vi "psp_zeromq_send.vi"(1 "socket out":refnum<class "zmq_socket.lvclass">, 2 "archive":T1) -> (0 "error out":errorcluster)   [LabVIEW 2020]
uses:
  <vilib>/addons/zeromq/zmq_socket.lvclass
  archive_elyse/archive.ctl
  archive_elyse/sync_type_def.ctl
  archive_elyse/HT_type-def.ctl
  archive_elyse/HF_type_def.ctl
  archive_elyse/vacuum_type_def.ctl
  archive_elyse/modulator_type_def.ctl
  archive_elyse/water_cooling_type_def.ctl
  archive_elyse/all_magnets_type_def.ctl
panel:
  out "JSON string":string
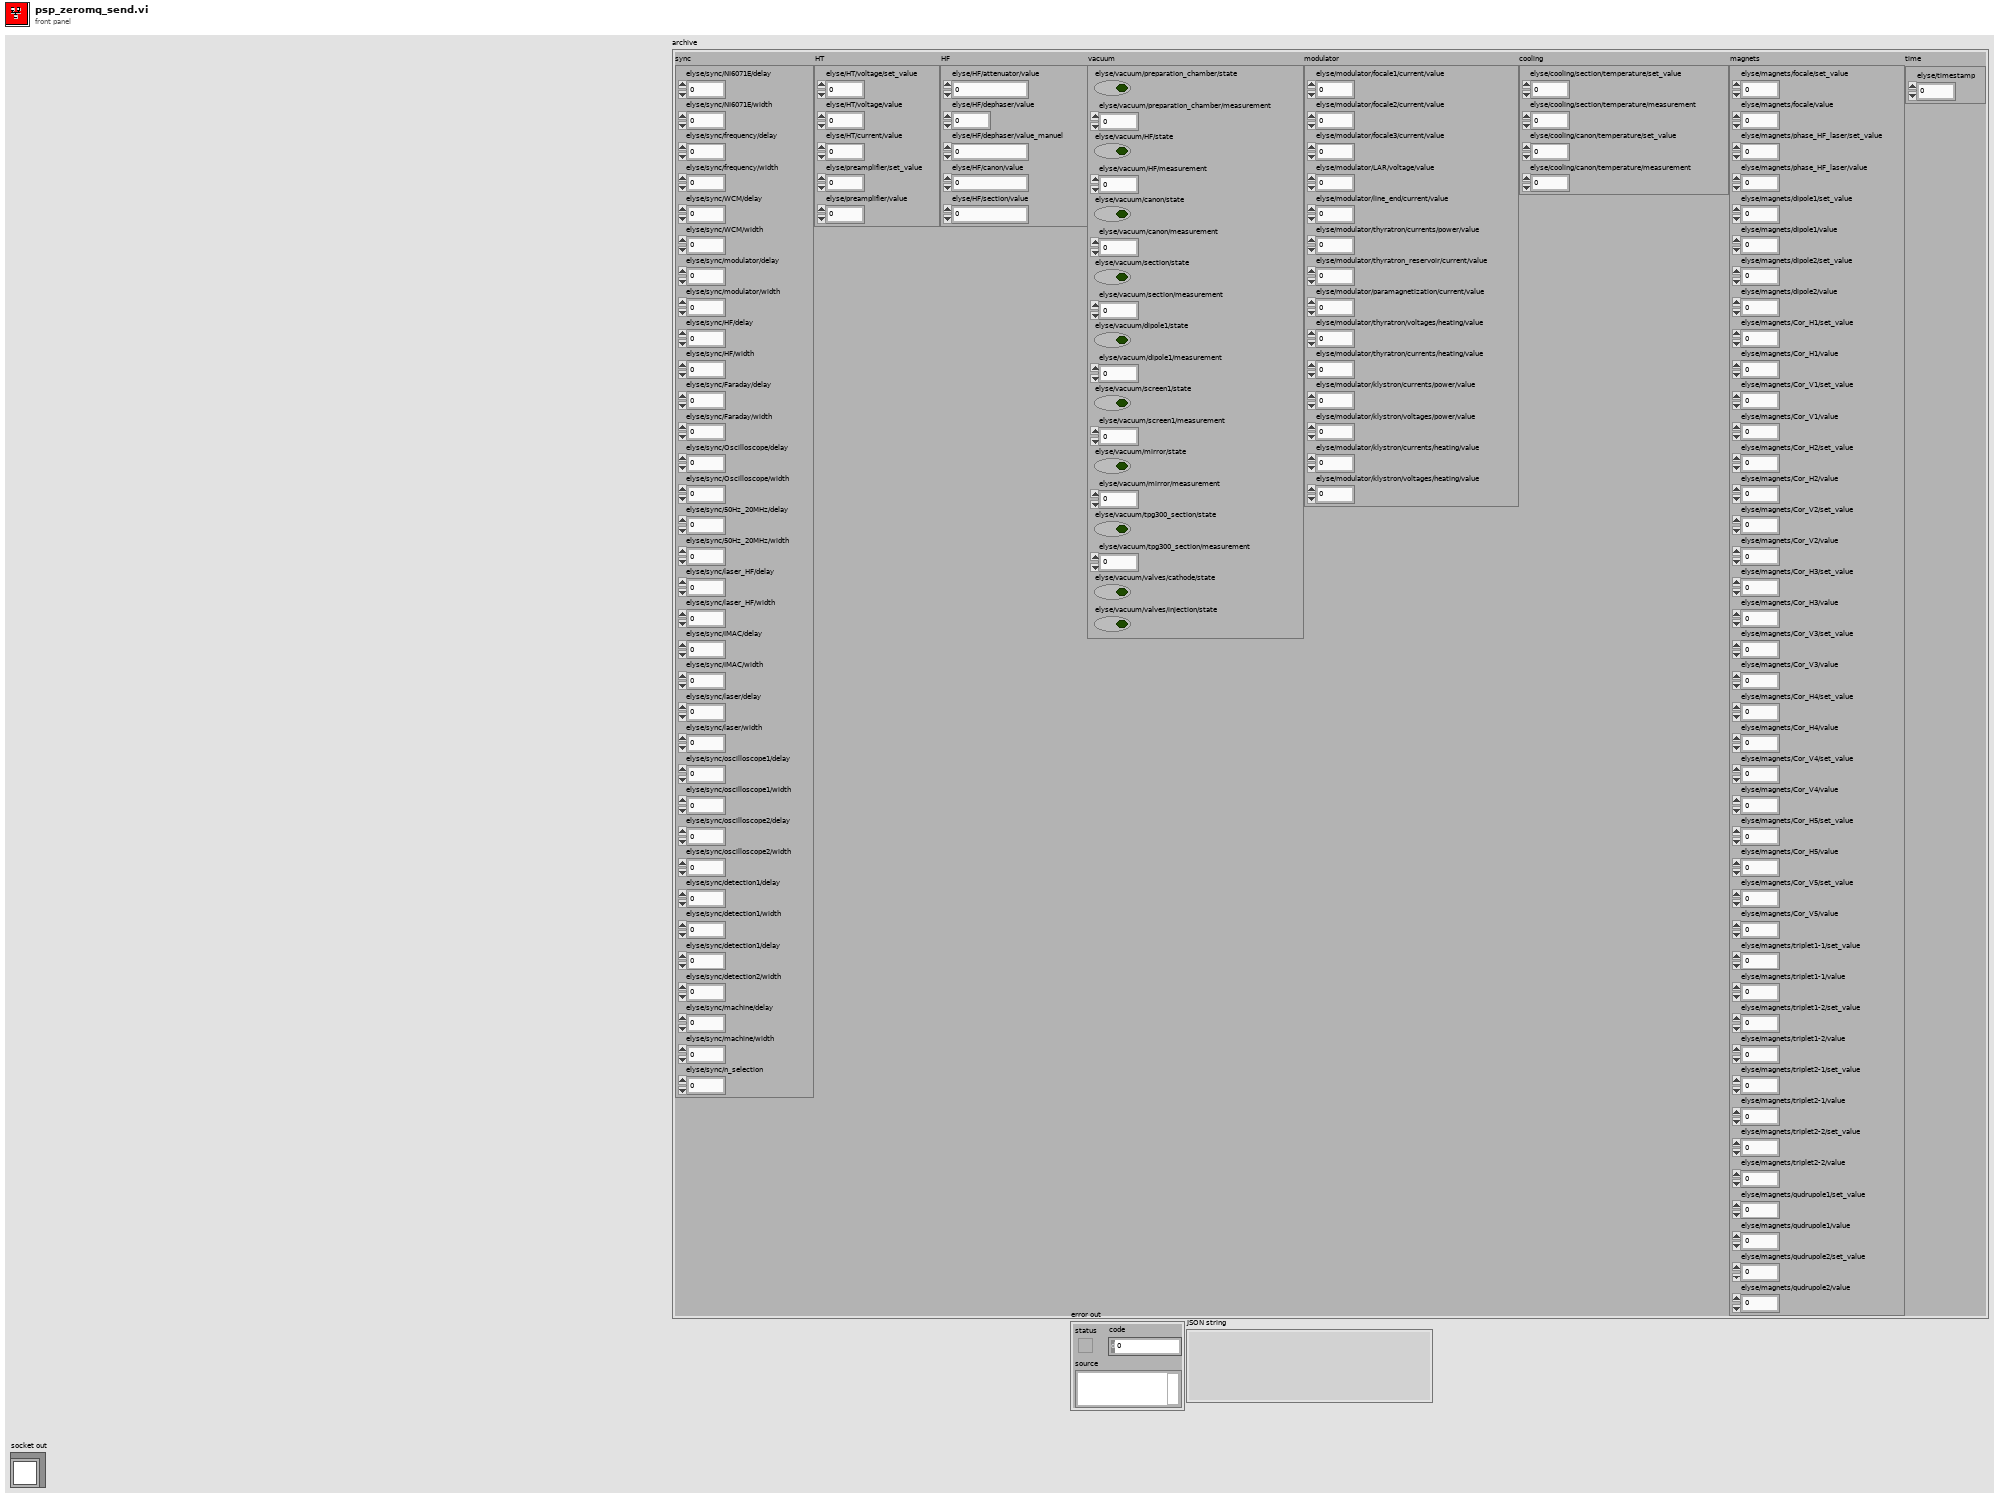
[diagram p1: front panel]
types:
  T1 = typedef "archive.ctl" = cluster{"sync":T2, "HT":T3, "HF":T4, "vacuum":T5, "modulator":T6, "cooling":T7, "magnets":T8, "time":cluster{"elyse/timestamp":dbl}}
  T2 = typedef "sync_type_def.ctl" = cluster{"elyse/sync/NI6071E/delay":dbl, "elyse/sync/NI6071E/width":dbl, "elyse/sync/frequency/delay":dbl, "elyse/sync/frequency/width":dbl, "elyse/sync/WCM/delay":dbl, "elyse/sync/WCM/width":dbl, "elyse/sync/modulator/delay":dbl, "elyse/sync/modulator/width":dbl, "elyse/sync/HF/delay":dbl, "elyse/sync/HF/width":dbl, "elyse/sync/Faraday/delay":dbl, "elyse/sync/Faraday/width":dbl, "elyse/sync/Oscilloscope/delay":dbl, "elyse/sync/Oscilloscope/width":dbl, "elyse/sync/50Hz_20MHz/delay":dbl, "elyse/sync/50Hz_20MHz/width":dbl, "elyse/sync/laser_HF/delay":dbl, "elyse/sync/laser_HF/width":dbl, "elyse/sync/IMAC/delay":dbl, "elyse/sync/IMAC/width":dbl, "elyse/sync/laser/delay":dbl, "elyse/sync/laser/width":dbl, "elyse/sync/oscilloscope1/delay":dbl, "elyse/sync/oscilloscope1/width":dbl, "elyse/sync/oscilloscope2/delay":dbl, "elyse/sync/oscilloscope2/width":dbl, "elyse/sync/detection1/delay":dbl, "elyse/sync/detection1/width":dbl, "elyse/sync/detection1/delay":dbl, "elyse/sync/detection2/width":dbl, "elyse/sync/machine/delay":dbl, "elyse/sync/machine/width":dbl, "elyse/sync/n_selection":dbl}
  T3 = typedef "HT_type-def.ctl" = cluster{"elyse/HT/voltage/set_value":dbl, "elyse/HT/voltage/value":dbl, "elyse/HT/current/value":dbl, "elyse/preamplifier/set_value":dbl, "elyse/preamplifier/value":dbl}
  T4 = typedef "HF_type_def.ctl" = cluster{"elyse/HF/attenuator/value":dbl, "elyse/HF/dephaser/value":dbl, "elyse/HF/dephaser/value_manuel":dbl, "elyse/HF/canon/value":dbl, "elyse/HF/section/value":dbl}
  T5 = typedef "vacuum_type_def.ctl" = cluster{"elyse/vacuum/preparation_chamber/state":bool, "elyse/vacuum/preparation_chamber/measurement":dbl, "elyse/vacuum/HF/state":bool, "elyse/vacuum/HF/measurement":dbl, "elyse/vacuum/canon/state":bool, "elyse/vacuum/canon/measurement":dbl, "elyse/vacuum/section/state":bool, "elyse/vacuum/section/measurement":dbl, "elyse/vacuum/dipole1/state":bool, "elyse/vacuum/dipole1/measurement":dbl, "elyse/vacuum/screen1/state":bool, "elyse/vacuum/screen1/measurement":dbl, "elyse/vacuum/mirror/state":bool, "elyse/vacuum/mirror/measurement":dbl, "elyse/vacuum/tpg300_section/state":bool, "elyse/vacuum/tpg300_section/measurement":dbl, "elyse/vacuum/valves/cathode/state":bool, "elyse/vacuum/valves/injection/state":bool}
  T6 = typedef "modulator_type_def.ctl" = cluster{"elyse/modulator/focale1/current/value":dbl, "elyse/modulator/focale2/current/value":dbl, "elyse/modulator/focale3/current/value":dbl, "elyse/modulator/LAR/voltage/value":dbl, "elyse/modulator/line_end/current/value":dbl, "elyse/modulator/thyratron/currents/power/value":dbl, "elyse/modulator/thyratron_reservoir/current/value":dbl, "elyse/modulator/paramagnetization/current/value":dbl, "elyse/modulator/thyratron/voltages/heating/value":dbl, "elyse/modulator/thyratron/currents/heating/value":dbl, "elyse/modulator/klystron/currents/power/value":dbl, "elyse/modulator/klystron/voltages/power/value":dbl, "elyse/modulator/klystron/currents/heating/value":dbl, "elyse/modulator/klystron/voltages/heating/value":dbl}
  T7 = typedef "water_cooling_type_def.ctl" = cluster{"elyse/cooling/section/temperature/set_value":dbl, "elyse/cooling/section/temperature/measurement":dbl, "elyse/cooling/canon/temperature/set_value":dbl, "elyse/cooling/canon/temperature/measurement":dbl}
  T8 = typedef "all_magnets_type_def.ctl" = cluster{"elyse/magnets/focale/set_value":dbl, "elyse/magnets/focale/value":dbl, "elyse/magnets/phase_HF_laser/set_value":dbl, "elyse/magnets/phase_HF_laser/value":dbl, "elyse/magnets/dipole1/set_value":dbl, "elyse/magnets/dipole1/value":dbl, "elyse/magnets/dipole2/set_value":dbl, "elyse/magnets/dipole2/value":dbl, "elyse/magnets/Cor_H1/set_value":dbl, "elyse/magnets/Cor_H1/value":dbl, "elyse/magnets/Cor_V1/set_value":dbl, "elyse/magnets/Cor_V1/value":dbl, "elyse/magnets/Cor_H2/set_value":dbl, "elyse/magnets/Cor_H2/value":dbl, "elyse/magnets/Cor_V2/set_value":dbl, "elyse/magnets/Cor_V2/value":dbl, "elyse/magnets/Cor_H3/set_value":dbl, "elyse/magnets/Cor_H3/value":dbl, "elyse/magnets/Cor_V3/set_value":dbl, "elyse/magnets/Cor_V3/value":dbl, "elyse/magnets/Cor_H4/set_value":dbl, "elyse/magnets/Cor_H4/value":dbl, "elyse/magnets/Cor_V4/set_value":dbl, "elyse/magnets/Cor_V4/value":dbl, "elyse/magnets/Cor_H5/set_value":dbl, "elyse/magnets/Cor_H5/value":dbl, "elyse/magnets/Cor_V5/set_value":dbl, "elyse/magnets/Cor_V5/value":dbl, "elyse/magnets/triplet1-1/set_value":dbl, "elyse/magnets/triplet1-1/value":dbl, "elyse/magnets/triplet1-2/set_value":dbl, "elyse/magnets/triplet1-2/value":dbl, "elyse/magnets/triplet2-1/set_value":dbl, "elyse/magnets/triplet2-1/value":dbl, "elyse/magnets/triplet2-2/set_value":dbl, "elyse/magnets/triplet2-2/value":dbl, "elyse/magnets/qudrupole1/set_value":dbl, "elyse/magnets/qudrupole1/value":dbl, "elyse/magnets/qudrupole2/set_value":dbl, "elyse/magnets/qudrupole2/value":dbl}
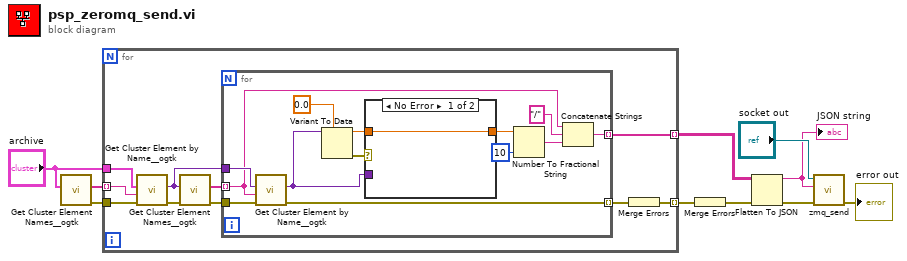
[diagram p0: block diagram]
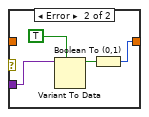
[diagram p2: hidden frame]
diagram:
  n1 = call <userlib>:"Get Cluster Element Names__ogtk.vi"("Cluster"="archive") -> ("error out"=w9:errorcluster, "Element Names"=w8:string[])  [unwired: 9 in]
  n2 = for {
    tunnel: w8 -> [w15] mode=indexing
    tunnel: "archive" -> [w20]
    tunnel: w9 -> [w18]
    tunnel: [w14] -> w7 mode=indexing
    tunnel: [w11] -> w4 mode=indexing
    n3 = call <userlib>:"Get Cluster Element by Name__ogtk.vi"("error in (no error)"=w18, "Element Name"=w15, "Cluster"=w20) -> ("error out"=w19:errorcluster, "VElement"=w16:variant)  [unwired: 6 in, 1 out]
    n4 = call <userlib>:"Get Cluster Element Names__ogtk.vi"("error in (no error)"=w19, "Cluster"=w16) -> ("error out"=w13:errorcluster, "Element Names"=w17:string[])  [unwired: 8 in]
    n5 = for {
      tunnel: w17 -> [w27] mode=indexing
      tunnel: w16 -> [w32]
      tunnel: [w26] -> w14 mode=indexing
      tunnel: w13 -> [w25]
      tunnel: [w24] -> w12 mode=indexing
      n6 = call <userlib>:"Get Cluster Element by Name__ogtk.vi"("error in (no error)"=w25, "Element Name"=w27, "Cluster"=w32) -> ("error out"=w24:errorcluster, "VElement"=w30:variant)  [unwired: 6 in, 1 out]
      n7 = Variant To Data(type=0.0, Variant=w30) -> (data=w29:dbl, error out=w31:errorcluster)  [unwired: 1 in]
      n8 = case shown="No Error" w31 {
        tunnel: w30 -> [_ w38]
        tunnel: [w34 w35] -> w28
        tunnel: w29 -> [w34 _]
        frame No Error {
        }
        frame Error {
          n9 = Variant To Data(type=TRUE, Variant=w38) -> (data=w36:bool)  [unwired: 1 in, 1 out]
          n10 = Boolean To (0,1)(Boolean=w36) -> (0, 1=w35:i16)
        }
      }
      n11 = Number To Fractional String(number=w28, precision (6)=i16 10) -> (F-format string=w23:string)  [unwired: 2 in]
      n12 = Concatenate Strings(w27, "/" ("string"), w23) -> (w26:string)
    }
    n13 = Merge Errors(w12) -> (w11:errorcluster)
  }
  n14 = Merge Errors(w4) -> (w3:errorcluster)
  n15 = Flatten To JSON(anything=w7, error in (no error)=w3) -> (JSON string=w6:string, 11:w2:errorcluster)  [unwired: 1 in]
  "JSON string" <- w6
  n16 = call <vilib>:"zmq_send.vi"("error in"=w2, "data"=w6, "socket in"="socket out") -> ("error out"=→"error out":errorcluster)  [unwired: 4 in, 1 out]
